vi "Is Indicator.vi"(11 "Indicator in":refnum<class "Indicator.lvclass">) -> (2 "Indicator":bool)   [LabVIEW 2020, in "VolatusGUI.lvlib" / "Indicator.lvclass"]
uses:
  Indicator.lvclass
  Indicator.lvclass/Indicator.ctl
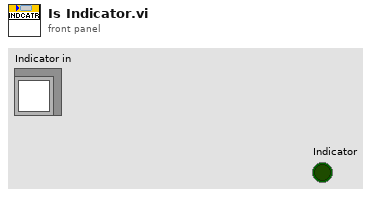
[diagram p1: front panel]
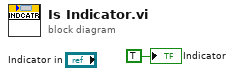
[diagram p0: block diagram]
diagram:
  "Indicator" <- TRUE ("Indicator")
